vi "WPI_CameraSendMarkedString.vi"(9 "timeout for TCP write":i32=1000, 10 "Data String":string, 11 "TCP Network Connection in":refnum<k5>) -> (0 "error out":errorcluster, 3 "TCP Network Connection out":refnum<k5>)   [LabVIEW 2017]
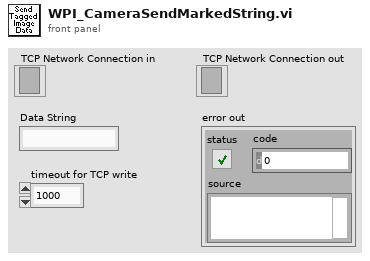
[diagram p1: front panel]
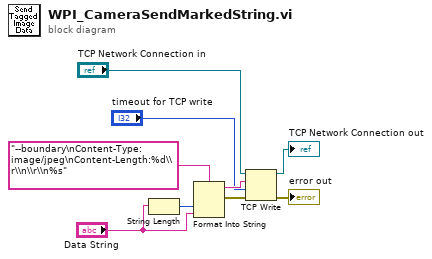
[diagram p0: block diagram]
diagram:
  n1 = String Length(string="Data String") -> (length=w3:i32)
  n2 = Format Into String(format string="--boundary\nContent-Type: image/jpeg\nContent-Length:%d\\r\\n\\r\\n%s" ("regular expression"), w3, "Data String") -> (resulting string=w6:string, error out=w5:errorcluster)  [unwired: 2 in]
  n3 = TCP Write(connection ID="TCP Network Connection in", data in=w6, error in (no error)=w5, 9:"timeout for TCP write") -> (connection ID out=→"TCP Network Connection out":refnum<k5>, error out=→"error out":errorcluster)  [unwired: 1 out]
